vi "CANOpen_Send NMT.vi"(6 "Init check":bool, 7 "Nodes":T2[](array[typedef]) {"NMT"."Node init static SDO state" items=["start remote node"=1, "enter pre-operational"=128]; "NMT"."Node run state" items=["start remote node"=1, "stop remote node"=2, "enter pre-operational"=128, "reset node"=129, "reset communication"=130]; "Dynamic SDOs"."Sub-Index (0)" format="%.0x"; "Dynamic SDOs"."Object Index" format="%.0x"; "Dynamic SDOs"."Block Data" format="%.0x"; "RPDOs"."PDO Channel" items=["PDO 1", "PDO 2", "PDO 3", "PDO 4"]; "RPDOs"."Parameters"."Bit Offset" max=8 step=1; "RPDOs"."Parameters"."Byte Offset" max=8 step=1; "TPDOs"."PDO Channel" items=["PDO 1", "PDO 2", "PDO 3", "PDO 4"]; "TPDOs"."Parameters"."Bit Offset" max=8 step=1; "TPDOs"."Parameters"."Byte Offset" max=8 step=1; "SDOs"."Sub-Index (0)" format="%.0x"; "SDOs"."Object Index" format="%.0x"; "SDOs"."Block Data" format="%.0x"}, 8 "error in":errorcluster, 9 "Security Ref in":T1, 10 "FIFO":refnum<k33>, 11 "interface object":refnum<k20>) -> (0 "error out":errorcluster, 1 "Security Ref out":T1, 2 "Node IDs to Check":i16[](array[numeric]), 3 "interface object out":refnum<k20>)   [LabVIEW 2013, in "CANOpen Addon Custom Device.lvlib"]
uses:
  CANOpen Addon Custom Device.lvlib
  CANOpen_Node Message Settings.ctl
  Shared Code/CANOpen_PDO Settings.ctl
  Shared Code/CANOpen_PDO Parameter Settings.ctl
  Shared Code/CANOpen_PDO Data Type.ctl
  System Explorer/SubVIs/CANopen Byte Order.ctl
  Shared Code/CANOpen_SDO Settings.ctl
  CANOpen_NMT Settings.ctl
  Async VIs/CANOpen_Main/SubVIs/CanOpen_NMT_Config.ctl
  Async VIs/CANOpen_Main/SubVIs/CanOpen_NMT_Static detect.ctl
  Async VIs/CANOpen_Main/SubVIs/CANOpen_HB_NG_EM Refs.ctl
  <vilib>/CANopenLib/CANOPEN.llb/CANopen Node Guarding Create.vi
  <vilib>/CANopenLib/CANOPEN.llb/CANopen Node Guarding Close.vi
  <vilib>/CANopenLib/CANOPEN.llb/CANopen Heartbeat Create.vi
  <vilib>/CANopenLib/CANOPEN.llb/CANopen Heartbeat Close.vi
  <vilib>/NI Veristand/Custom Device Tools/Custom Device Utility Library/Custom Device Utility Library.lvlib
  <resource>/objmgr/CANopenHeartbeat.rc
  <resource>/objmgr/CANopenNodeGuard.rc
panel:
  # "LSB"
  # "MSB"
  # "LSB"
  # "MSB"
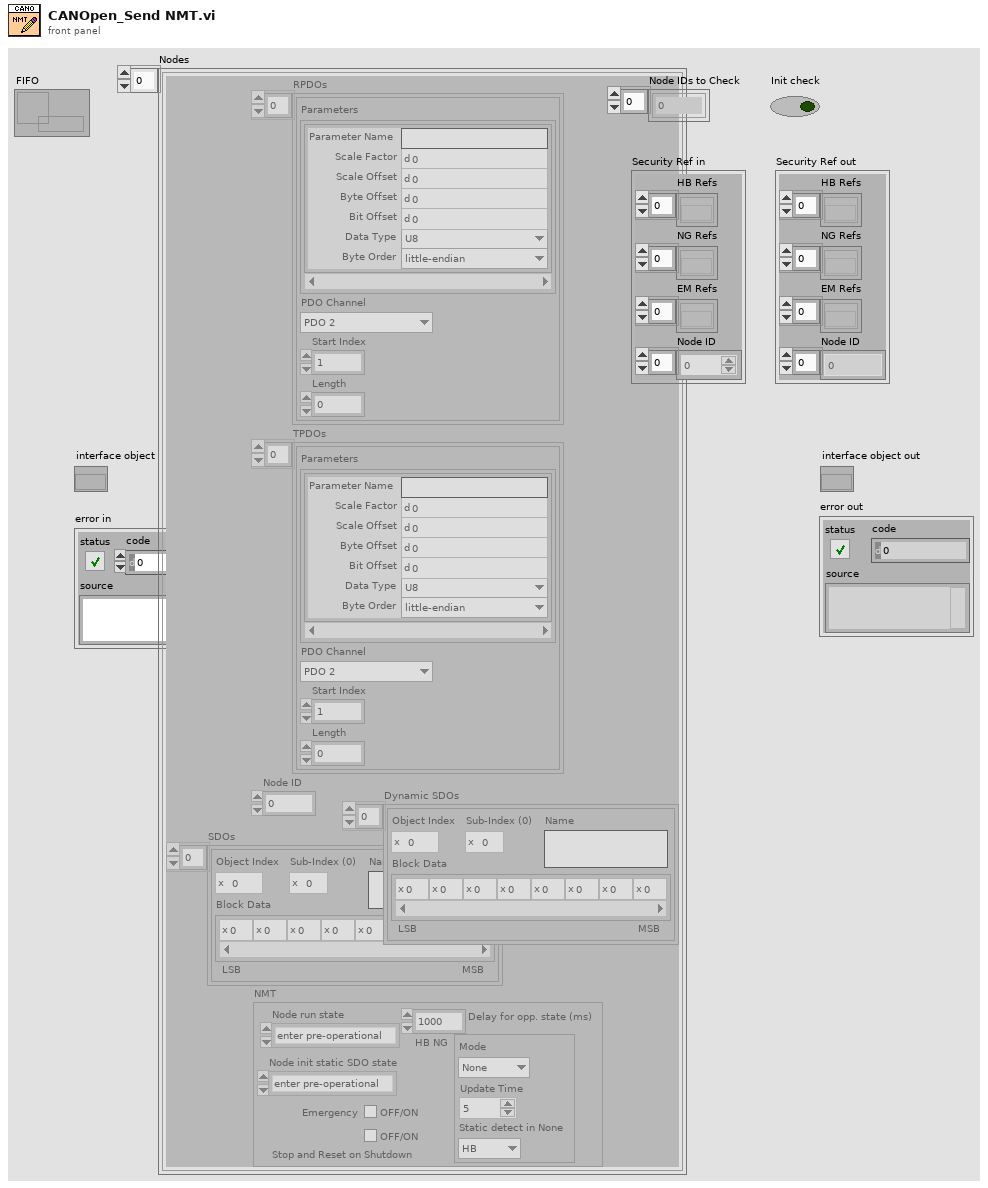
[diagram p1: front panel]
types:
  T1 = typedef "CANOpen Addon Custom Device.lvlib/CANOpen_HB_NG_EM Refs.ctl" = cluster{"HB Refs":refnum<k20>[], "NG Refs":refnum<k20>[], "EM Refs":refnum<k20>[], "Node ID":u8[]}
  T2 = typedef "CANOpen_Node Message Settings.ctl" = cluster{"RPDOs":T3[], "TPDOs":T3[], "Node ID":u8, "SDOs":T7[], "Dynamic SDOs":T7[], "NMT":T8}
  T3 = typedef "CANOpen Addon Custom Device.lvlib/CANOpen_PDO Settings.ctl" = cluster{"Parameters":T4[], "PDO Channel":u8, "Start Index":u32, "Length":u32}
  T4 = typedef "CANOpen Addon Custom Device.lvlib/CANOpen_PDO Parameter Settings.ctl" = cluster{"Parameter Name":string, "Scale Factor":dbl, "Scale Offset":dbl, "Byte Offset":u8, "Bit Offset":u8, "Data Type":T5, "Byte Order":T6}
  T5 = typedef "CANOpen Addon Custom Device.lvlib/CANOpen_PDO Data Type.ctl" = enum16{"U8", "U16", "U32", "I8", "I16", "I32", "Single", "Double", "Boolean"}
  T6 = typedef "CANOpen Addon Custom Device.lvlib/CANopen Byte Order.ctl" = enum16{"big-endian network order", "little-endian"}
  T7 = typedef "CANOpen Addon Custom Device.lvlib/CANOpen_SDO Settings.ctl" = cluster{"Object Index":u16, "Sub-Index (0)":u8, "Block Data":u8[], "Name":string}
  T8 = typedef "CANOpen Addon Custom Device.lvlib/CANOpen_NMT Settings.ctl" = cluster{"Node run state":u16, "Emergency":bool, "HB NG":T9, "Delay for opp. state (ms)":dbl, "Node init static SDO state":u16, "Stop and Reset on Shutdown":bool}
  T9 = typedef "CANOpen Addon Custom Device.lvlib/CanOpen_NMT_Config.ctl" = cluster{"Mode":T10, "Update Time":u16, "Static detect in None":T10}
  T10 = typedef "CANOpen Addon Custom Device.lvlib/CanOpen_NMT_Static detect.ctl" = enum16{"None", "HB", "NG"}
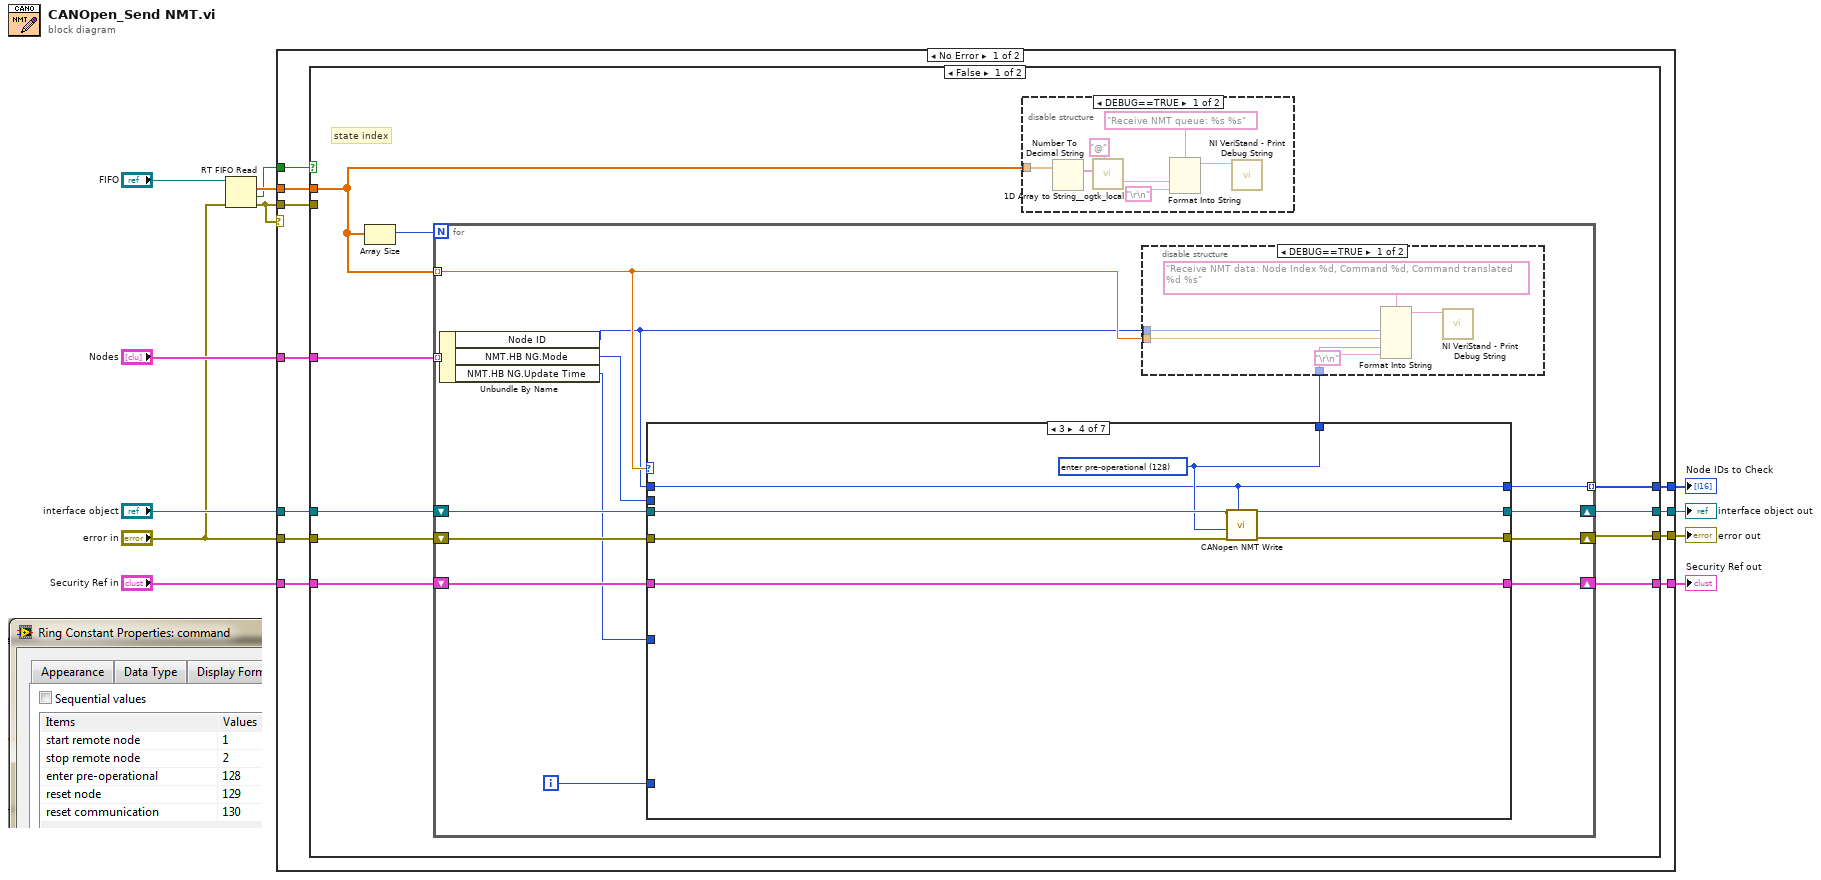
[diagram p0: block diagram]
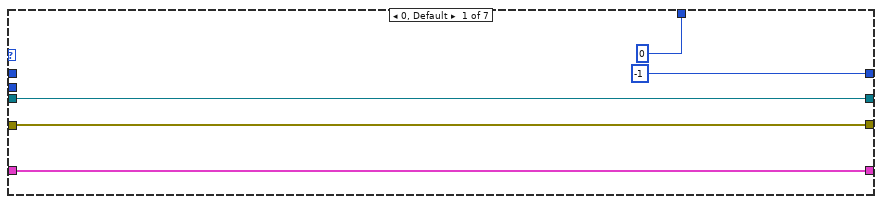
[diagram p2: hidden frame]
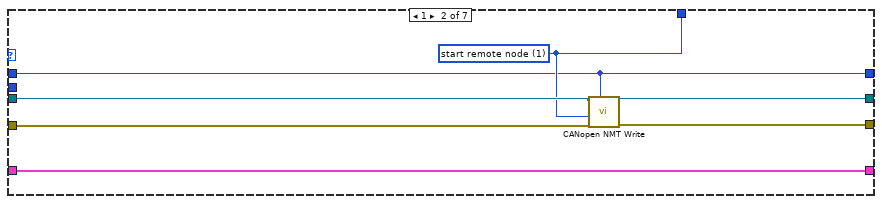
[diagram p3: hidden frame]
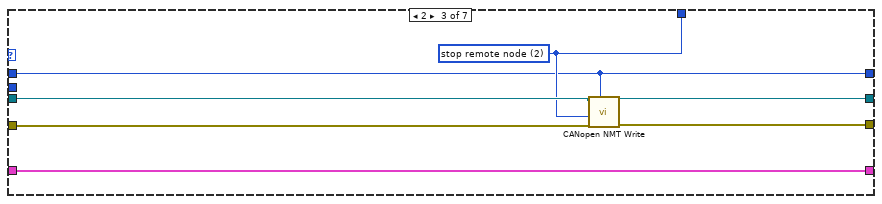
[diagram p4: hidden frame]
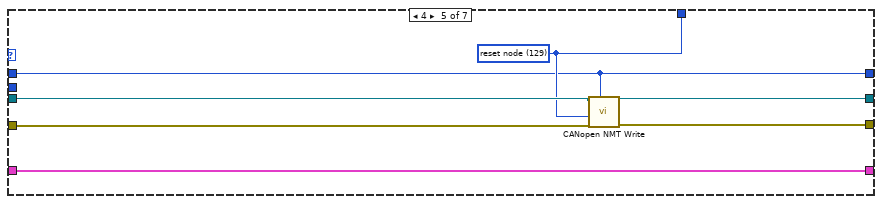
[diagram p5: hidden frame]
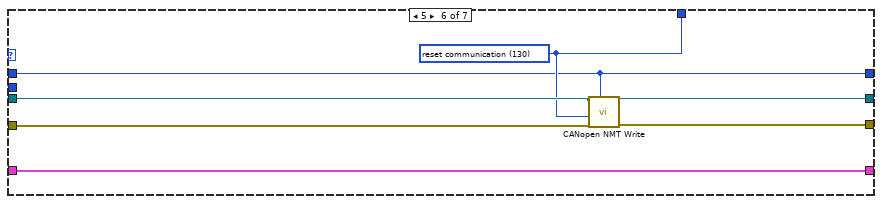
[diagram p6: hidden frame]
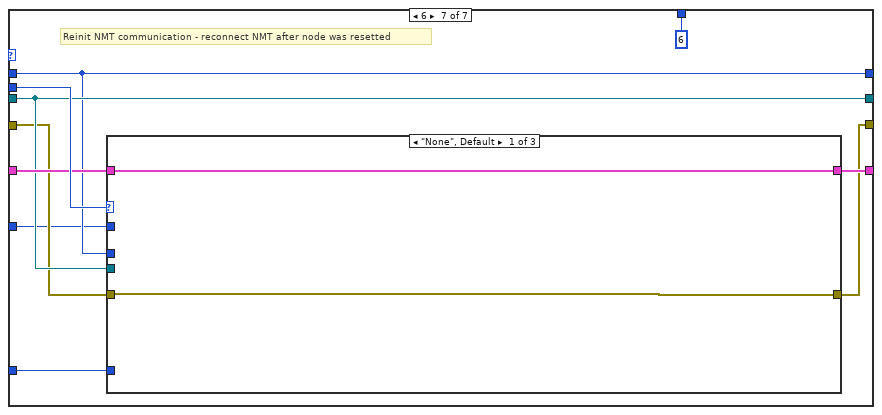
[diagram p7: hidden frame]
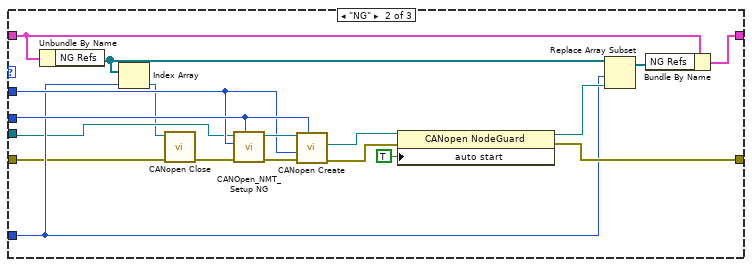
[diagram p8: hidden frame]
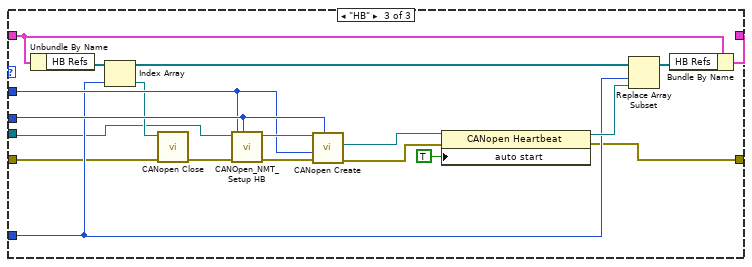
[diagram p9: hidden frame]
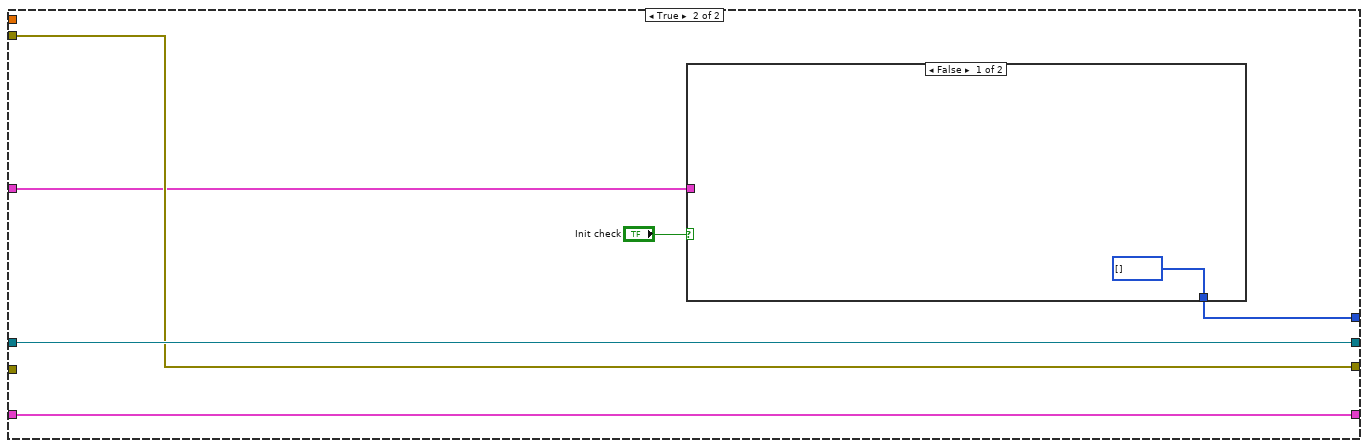
[diagram p12: hidden frame]
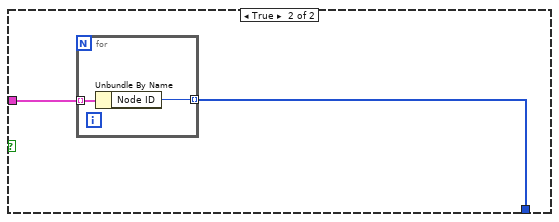
[diagram p13: hidden frame]
diagram:
  n1 = RT FIFO Read(0:"FIFO", 3:"error in") -> (9:w7:dbl[], 10:w6:bool, 11:w1:errorcluster)  [unwired: 2 in, 2 out]
  n2 = case shown="No Error" w1 {
    tunnel: "Nodes" -> [w23 _]
    tunnel: "interface object" -> [w22 w162]
    tunnel: w1 -> [w21 _]
    tunnel: [w20 w161] -> w9
    tunnel: [w19 w162] -> w8
    tunnel: w7 -> [w18 _]
    tunnel: w6 -> [w17 _]
    tunnel: "error in" -> [w16 w161]
    tunnel: [w15 _] -> w4
    tunnel: "Security Ref in" -> [w14 w160]
    tunnel: [w13 w160] -> w2
    frame No Error {
      n3 = case shown="False" w17 {
        tunnel: w23 -> [w33 w149]
        tunnel: w22 -> [w31 w154]
        tunnel: w21 -> [_ w153]
        tunnel: [w29 w153] -> w20
        tunnel: [w32 w154] -> w19
        tunnel: w18 -> [w27 _]
        tunnel: w16 -> [w30 _]
        tunnel: [w28 w152] -> w15
        tunnel: w14 -> [w25 w151]
        tunnel: [w24 w151] -> w13
        frame False {
          # "state index"
          n4 = Array Size(array=w27) -> (size(s)=w26:i32)
          n5 = for {
            N: w26 -> [_]
            tunnel: w33 -> [w43] mode=indexing
            tunnel: w27 -> [w42] mode=indexing
            shift-right: [w47] -> w32
            shift-left: w31 -> [w45]
            shift-right: [w44] -> w29
            shift-left: w30 -> [w46]
            tunnel: [w34] -> w28 mode=indexing
            shift-right: [w37] -> w24
            shift-left: w25 -> [w40]
            i -> [w39]
            n6 = Unbundle By Name(w43) -> ("Node ID"=w35:u8, "NMT.HB NG.Mode"=w38:T10, "NMT.HB NG.Update Time"=w36:u16)
            n7 = case shown="3" w42 {
              tunnel: [w52 w59 w66 w73 w80 w87 w93] -> w47
              tunnel: w46 -> [w51 w58 w65 w72 w79 w86 w91]
              tunnel: w45 -> [w52 w57 w64 w71 w78 w85 w93]
              tunnel: [w51 w56 w63 w70 w77 w84 w90] -> w44
              tunnel: w35 -> [_ w54 w61 w68 w75 w82 w92]
              tunnel: [u16 0 ("command") w55 w62 w69 w76 w83 u16 6 ("command")] -> w41
              tunnel: [i16 -1 ("Node ID") w54 w61 w68 w75 w82 w92] -> w34
              tunnel: w40 -> [w48 w53 w60 w67 w74 w81 w94]
              tunnel: w39 -> [_ _ _ _ _ _ w89]
              tunnel: w38 -> [_ _ _ _ _ _ w96]
              tunnel: [w48 w53 w60 w67 w74 w81 w95] -> w37
              tunnel: w36 -> [_ _ _ _ _ _ w88]
              frame 0, Default {
              }
              frame 1 {
                w55 = u16 1 items=["start remote node"=1, "stop remote node"=2, "enter pre-operational"=128, "reset node"=129, "reset communication"=130] ("command")
                n8 = call <vilib>:"CANopen NMT Write.vi"("node-ID (0)"=w54, "error in (no error)"=w58, "command"=w55, "interface object in"=w57) -> ("error out"=w56:errorcluster, "interface object out"=w59:refnum<k20>)  [unwired: 6 in]
              }
              frame 2 {
                w62 = u16 2 items=["start remote node"=1, "stop remote node"=2, "enter pre-operational"=128, "reset node"=129, "reset communication"=130] ("command")
                n9 = call <vilib>:"CANopen NMT Write.vi"("node-ID (0)"=w61, "error in (no error)"=w65, "command"=w62, "interface object in"=w64) -> ("error out"=w63:errorcluster, "interface object out"=w66:refnum<k20>)  [unwired: 6 in]
              }
              frame 3 {
                w69 = u16 128 items=["start remote node"=1, "stop remote node"=2, "enter pre-operational"=128, "reset node"=129, "reset communication"=130] ("command")
                n10 = call <vilib>:"CANopen NMT Write.vi"("node-ID (0)"=w68, "error in (no error)"=w72, "command"=w69, "interface object in"=w71) -> ("error out"=w70:errorcluster, "interface object out"=w73:refnum<k20>)  [unwired: 6 in]
              }
              frame 4 {
                w76 = u16 129 items=["start remote node"=1, "stop remote node"=2, "enter pre-operational"=128, "reset node"=129, "reset communication"=130] ("command")
                n11 = call <vilib>:"CANopen NMT Write.vi"("node-ID (0)"=w75, "error in (no error)"=w79, "command"=w76, "interface object in"=w78) -> ("error out"=w77:errorcluster, "interface object out"=w80:refnum<k20>)  [unwired: 6 in]
              }
              frame 5 {
                w83 = u16 130 items=["start remote node"=1, "stop remote node"=2, "enter pre-operational"=128, "reset node"=129, "reset communication"=130] ("command")
                n12 = call <vilib>:"CANopen NMT Write.vi"("node-ID (0)"=w82, "error in (no error)"=w86, "command"=w83, "interface object in"=w85) -> ("error out"=w84:errorcluster, "interface object out"=w87:refnum<k20>)  [unwired: 6 in]
              }
              frame 6 {
                # "Reinit NMT communication - reconnect NMT after node was resetted"
                n13 = case shown="\"None\", Default" w96 {
                  tunnel: [w99 w110 w132] -> w95
                  tunnel: w94 -> [w99 w109 w131]
                  tunnel: w93 -> [_ w103 w118]
                  tunnel: w92 -> [_ w115 w126]
                  tunnel: [w98 w111 w122] -> w90
                  tunnel: w91 -> [w98 w102 w121]
                  tunnel: w89 -> [_ w104 w123]
                  tunnel: w88 -> [_ w106 w125]
                  frame "None", Default {
                  }
                  frame "NG" {
                    n14 = Unbundle By Name(w109) -> ("NG Refs"=w105:refnum<k20>[])
                    n15 = Index Array(array=w105, index=w104) -> (element=w100:refnum<k20>)
                    n16 = call-poly <vilib>:"CANopen Close.vi"("error in (no error)"=w102, "node guarding object in"=w100) -> ("error out"=w101:errorcluster)  [unwired: 9 in]
                    n17 = call "CANOpen_NMT_Setup NG.vi"("Node ID"=w115, "error in"=w101, "Period"=w106, "interface object in"=w103) -> ("error out"=w116:errorcluster, "interface object out"=w117:refnum<k20>)  [unwired: 6 in]
                    n18 = call-poly <vilib>:"CANopen Create.vi"("node-ID"=w115, "error in (no error)"=w116, "guard time [ms]"=w106, "interface object in"=w117) -> ("error out"=w112:errorcluster, "node guarding object out"=w113:refnum<k20>)  [unwired: 5 in, 1 out]
                    n19 = property class="CANopen NodeGuard"(reference=w113, error in=w112, "auto start"=TRUE) -> (reference out=w107:refnum<k20>, error out=w111:errorcluster)
                    n20 = Replace Array Subset(array=w105, new element=w107, index=w104) -> (w108:refnum<k20>[])
                    n21 = Bundle By Name(cluster=w109, "NG Refs"=w108) -> (w110:T1)
                  }
                  frame "HB" {
                    n22 = Unbundle By Name(w131) -> ("HB Refs"=w124:refnum<k20>[])
                    n23 = Index Array(array=w124, index=w123) -> (element=w119:refnum<k20>)
                    n24 = call-poly <vilib>:"CANopen Close.vi"("error in (no error)"=w121, "heartbeat object in"=w119) -> ("error out"=w120:errorcluster)  [unwired: 9 in]
                    n25 = call "CANOpen_NMT_Setup HB.vi"("Node ID"=w126, "error in"=w120, "Period"=w125, "interface object in"=w118) -> ("error out"=w128:errorcluster, "interface object out"=w127:refnum<k20>)  [unwired: 6 in]
                    n26 = call-poly <vilib>:"CANopen Create.vi"("node-ID"=w126, "error in (no error)"=w128, "consumer time [ms]"=w125, "interface object in"=w127) -> ("error out"=w133:errorcluster, "heartbeat object out"=w134:refnum<k20>)  [unwired: 5 in, 1 out]
                    n27 = property class="CANopen Heartbeat"(reference=w134, error in=w133, "auto start"=TRUE) -> (reference out=w129:refnum<k20>, error out=w122:errorcluster)
                    n28 = Replace Array Subset(array=w124, new element=w129, index=w123) -> (w130:refnum<k20>[])
                    n29 = Bundle By Name(cluster=w131, "HB Refs"=w130) -> (w132:T1)
                  }
                }
              }
            }
            n30 = disable-structure shown="DEBUG==TRUE" {
              disable-tunnel: w35 -> [w139 _]
              disable-tunnel: w42 -> [w138 _]
              disable-tunnel: w41 -> [w137 _]
              frame condition #0 {
                n31 = Format Into String(format string="Receive NMT data: Node Index %d, Command %d, Command translated %d %s", w139, w138, w137, "\r\n") -> (resulting string=w140:string)  [unwired: 2 in, 1 out]
                n32 = call <vilib>:"NI VeriStand - Print Debug String.vi"("Message"=w140) -> ()  [unwired: 10 in, 1 out]
              }
              frame condition #1 (active) {
              }
            }
          }
          n33 = disable-structure shown="DEBUG==TRUE" {
            disable-tunnel: w27 -> [w146 _]
            frame condition #0 {
              n34 = Number To Decimal String(number=w146) -> (decimal integer string=w147:string[])  [unwired: 1 in]
              n35 = call "1D Array to String__ogtk_local.vi"("delimiter (Tab)"="@", "Array of Strings"=w147) -> ("delimited string"=w143:string)  [unwired: 9 in]
              n36 = Format Into String(format string="Receive NMT queue: %s %s", w143, "\r\n") -> (resulting string=w144:string)  [unwired: 2 in, 1 out]
              n37 = call <vilib>:"NI VeriStand - Print Debug String.vi"("Message"=w144) -> ()  [unwired: 10 in, 1 out]
            }
            frame condition #1 (active) {
            }
          }
        }
        frame True {
          n38 = case shown="False" "Init check" {
            tunnel: [u8[] [] w156] -> w152
            tunnel: w149 -> [_ w157]
            frame False {
            }
            frame True {
              n39 = for {
                tunnel: w157 -> [w159] mode=indexing
                tunnel: [w158] -> w156 mode=indexing
                n40 = Unbundle By Name(w159) -> ("Node ID"=w158:u8)
              }
            }
          }
        }
      }
    }
    frame Error {
    }
  }
  "error out" <- w9
  "interface object out" <- w8
  "Node IDs to Check" <- w4
  "Security Ref out" <- w2
